vi "New JSON Array (Numeric).vi"(8 "error in (no error)":errorcluster, 10 "Numeric Array":dbl[](array[numeric])) -> (0 "error out":errorcluster, 3 "JSON Value out":refnum<class "JSON Value.lvclass">)   [LabVIEW 2016, in "JSON Value.lvclass"]
doc: "bCreates a new JSON Array initialized with JSON Boolean objects of the values specified by Numeric Array"
uses:
  JSON Value.lvclass
  New JSON Numeric.vi
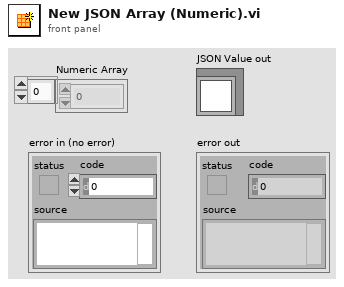
[diagram p1: front panel]
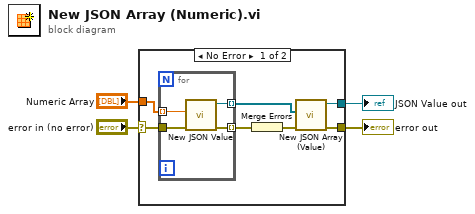
[diagram p0: block diagram]
diagram:
  n1 = case shown="No Error" "error in (no error)" {
    selector: "error in (no error)" -> [w8 w16]
    tunnel: [w5 w16] -> w3
    tunnel: [w9 _] -> w2
    tunnel: "Numeric Array" -> [w11 _]
    frame No Error {
      n2 = for {
        tunnel: w11 -> [w15] mode=indexing
        tunnel: [w14] -> w10 mode=indexing
        tunnel: w8 -> [w13]
        tunnel: [w12] -> w7 mode=indexing
        n3 = call-poly "New JSON Value.vi"("error in (no error)"=w13, "value"=w15) -> ("error out"=w12:errorcluster, "JSON Value out"=w14:refnum<class "JSON Value.lvclass">)  [unwired: 8 in]
      }
      n4 = Merge Errors(w7) -> (w6:errorcluster)
      n5 = call "New JSON Array (Value).vi"("error in (no error)"=w6, "JSON Datatypes"=w10) -> ("error out"=w5:errorcluster, "JSON Value out"=w9:refnum<class "JSON Value.lvclass">)  [unwired: 8 in]
    }
    frame Error {
    }
  }
  "error out" <- w3
  "JSON Value out" <- w2
